vi "TIO RPC Notification.vi"(5 "Timeout in ms":i32=1000, 7 "error in (no error)":errorcluster, 8 "Payload":string, 9 "Topic":string, 10 "TIO":T1={"TS Connection"={"Type"=enum."Serial", "URL"="serial:///dev/cu.usbserial-00000", "TO"=500, "Addr"=0, "Port"=0, "TCP"=refnum, "UDP"=refnum, "Route"=""}, "REQ"=refnum, "REP"=refnum}) -> (0 "error out":errorcluster, 1 "REP":string, 3 "Response":bool)   [LabVIEW 2010]
panel:
  out "timed out?":bool
  out "Topic 2":string
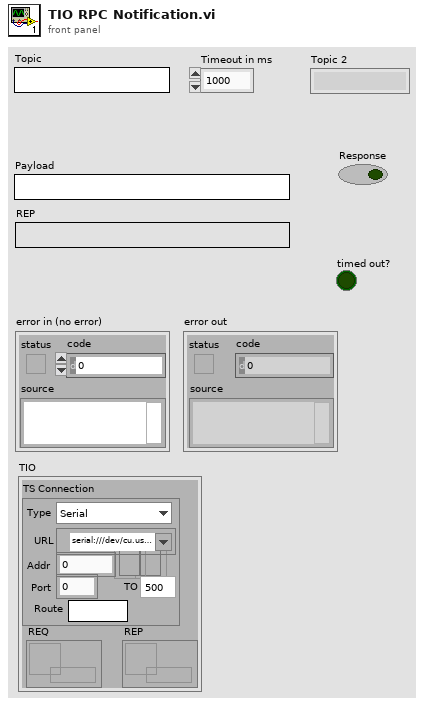
[diagram p1: front panel]
types:
  T1 = cluster{"TS Connection":cluster{"Type":enum16{"Serial", "TCP", "UDP", "mUDP"}, "URL":refnum<visa-resource-name>, "TO":u32, "Addr":u32, "Port":i32, "TCP":refnum<k5>, "UDP":refnum<k16>, "Route":string}, "REQ":refnum<queue>, "REP":refnum<queue>}
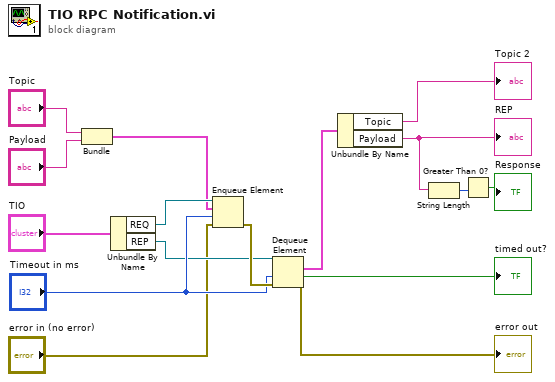
[diagram p0: block diagram]
diagram:
  n1 = Bundle("Topic"="Topic", "Payload"="Payload") -> (w1:cluster{"Topic":string, "Payload":string})  [unwired: 1 in]
  n2 = Unbundle By Name("TIO") -> ("REQ"=w7:refnum<queue>, "REP"=w6:refnum<queue>)
  n3 = Enqueue Element(queue=w7, element=w1, timeout in ms (-1)="Timeout in ms", error in (no error)="error in (no error)") -> (error out=w12:errorcluster)  [unwired: 2 out]
  n4 = Dequeue Element(queue=w6, timeout in ms (-1)="Timeout in ms", error in (no error)=w12) -> (element=w10:cluster{"Topic":string, "Payload":string}, timed out?=→"timed out?":bool, error out=→"error out":errorcluster)  [unwired: 1 out]
  n5 = Unbundle By Name(w10) -> ("Topic"=→"Topic 2":string, "Payload"=w15:string)
  "REP" <- w15
  n6 = String Length(string=w15) -> (length=w14:i32)
  n7 = Greater Than 0?(x=w14) -> (x > 0?=→"Response":bool)
